vi "UPDATE SQL ENG.vi"(9 "PRODUCTO":string, 10 "number":i32, 11 "TABLA":string) -> ()   [LabVIEW 2019]
uses:
  <vilib>/drjdpowell/SQLite Library/SQL Connection/Open (path).vi
  <vilib>/drjdpowell/SQLite Library/SQL Connection/Open (string).vi
  <vilib>/AdvancedString/Path To Command Line String.vi
  <vilib>/drjdpowell/SQLite Library/SQL Connection/Execute SQL (No results).vi
  <vilib>/drjdpowell/SQLite Library/SQL Connection/Connection.lvclass
  <vilib>/drjdpowell/SQLite Library/SQLite.lvlib
panel:
  out "concatenated string":string
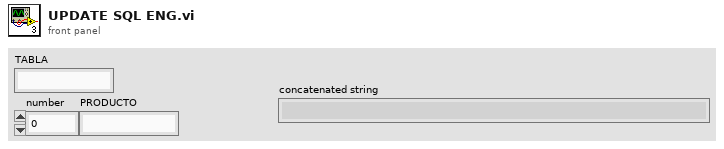
[diagram p1: front panel]
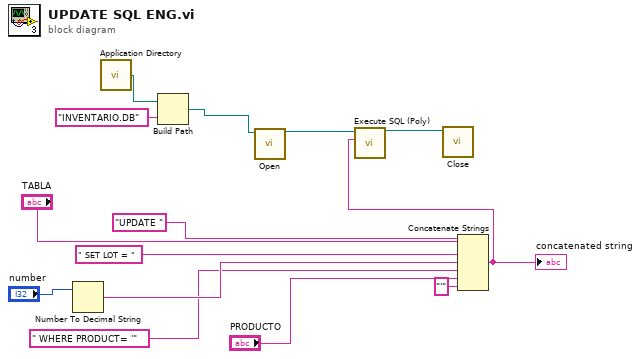
[diagram p0: block diagram]
diagram:
  n1 = Number To Decimal String(number="number") -> (decimal integer string=w10:string)  [unwired: 1 in]
  n2 = call <vilib>:"Application Directory.vi"() -> ("Application Directory"=w3:path)
  n3 = Build Path(base path=w3, name or relative path="INVENTARIO.DB") -> (appended path=w4:path)
  n4 = call-poly <vilib>:"Open.vi"("db file"=w4) -> ("SQLite Connection"=w5:refnum<class "Connection.lvclass">)  [unwired: 9 in, 1 out]
  n5 = Concatenate Strings("UPDATE " ("string"), "TABLA", " SET LOT = " ("string"), w10, " WHERE PRODUCT= '" ("string"), "PRODUCTO", "'" ("string")) -> (w1:string)
  "concatenated string" <- w1
  n6 = call-poly <vilib>:"Execute SQL (Poly).vi"("SQL"=w1, "SQLite Connection in"=w5) -> ("SQLite Connection"=w6:refnum<class "Connection.lvclass">)  [unwired: 8 in, 1 out]
  n7 = call-dynamic "Close.vi"("SQLite Connection in"=w6) -> ()  [unwired: 10 in, 1 out]
